vi "Event Log.vi"(8 "Message":string, 9 "Log Event Type":T1, 10 "Event Type":string, 11 "Location":string) -> ()   [LabVIEW 2024, in "Sift TDMS Uploader.lvlib" / "Sift TDMS Uploader.lvclass"]
uses:
  Sift TDMS Uploader.lvclass
  Sift TDMS Uploader.lvclass/Sift TDMS Uploader.ctl
  Log Event Types.ctl
panel:
  in  "error in (no error)":errorcluster
  out "error out":errorcluster
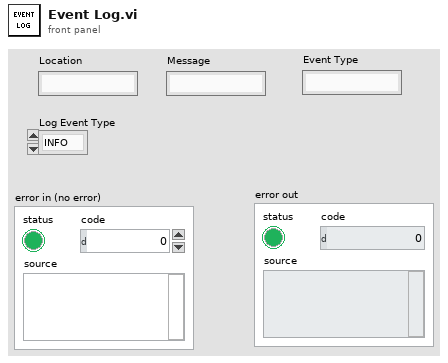
[diagram p1: front panel]
types:
  T1 = typedef "Sift TDMS Uploader.lvlib/Sift TDMS Uploader.lvclass/Log Event Types.ctl" = enum16{"INFO", "WARN", "ERROR"}
  T2 = enum16{"open", "replace", "create", "open or create", "replace or create", "replace or create with confirmation"}
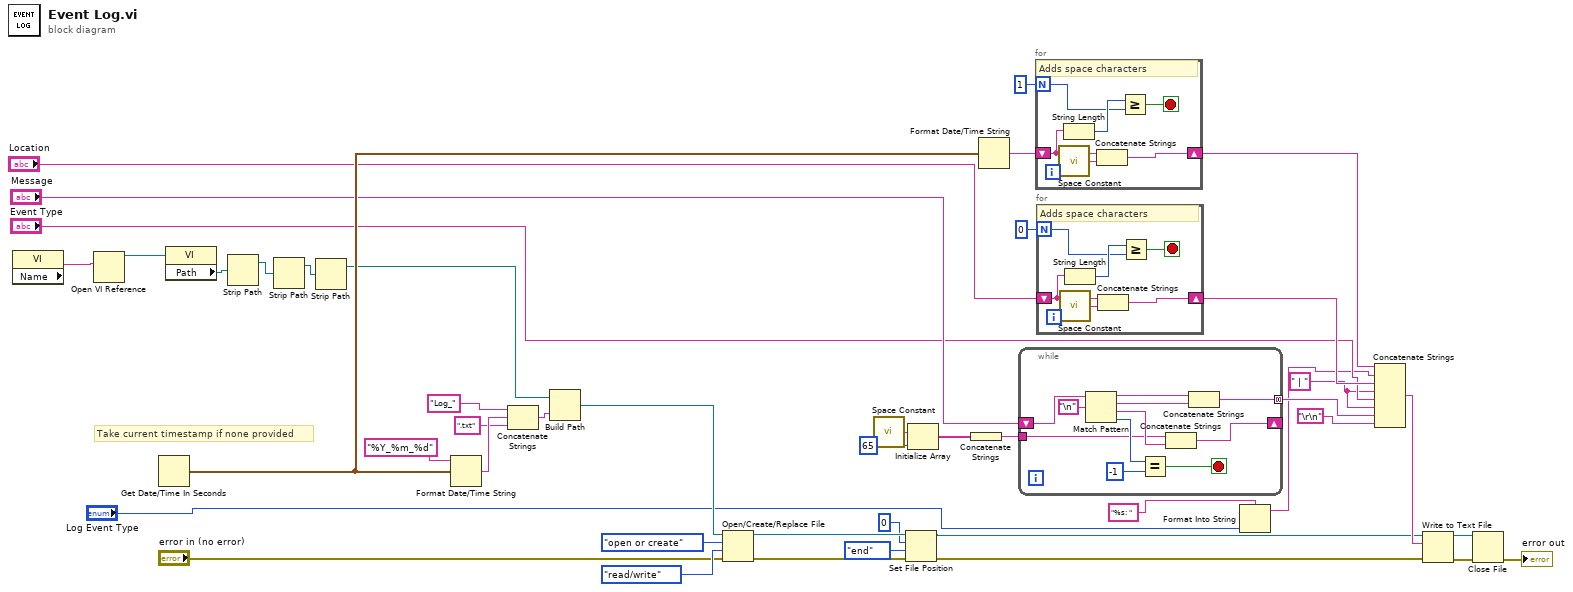
[diagram p0: block diagram]
diagram:
  w7 = " | " ("string")
  # "Take current timestamp if none provided"
  n1 = property class="VI"() -> ("Name"=w13:string)  [unwired: 2 in, 2 out]
  n2 = Open VI Reference(vi path=w13) -> (vi reference=w15:refnum<vi>)  [unwired: 5 in, 1 out]
  n3 = Get Date/Time In Seconds() -> (seconds since 1Jan1904=w17:timestamp)
  n4 = property class="VI"(reference=w15) -> ("Path"=w14:path)  [unwired: 1 in, 2 out]
  n5 = Strip Path(path=w14) -> (stripped path=w6:path)  [unwired: 1 out]
  n6 = Strip Path(path=w6) -> (stripped path=w2:path)  [unwired: 1 out]
  n7 = Strip Path(path=w2) -> (stripped path=w3:path)  [unwired: 1 out]
  n8 = Format Date/Time String(time format string (%c)="%Y_%m_%d", seconds (now)=w17) -> (date/time string=w32:string)  [unwired: 1 in]
  n9 = Concatenate Strings("Log_" ("string"), w32, ".txt" ("string")) -> (w31:string)
  n10 = Build Path(base path=w3, name or relative path=w31) -> (appended path=w18:path)
  n11 = Open/Create/Replace File(file path (use dialog)=w18, error in="error in (no error)", operation (0:open)=T2."open or create", access (0:read/write)=enum16{"read/write", "read-only", "write-only"}."read/write") -> (refnum out=w27:refnum<file>, error out=w28:errorcluster)  [unwired: 2 in, 1 out]
  n12 = call <vilib>:"Space Constant.vi"() -> ("String"=w38:string)
  n13 = Set File Position(offset (in bytes) (0)=i64 0, refnum=w27, from (0:start)=enum16{"start", "end", "current"}."end", error in=w28) -> (refnum out=w19:refnum<file>, error out=w23:errorcluster)
  n14 = Initialize Array(w38, 65 ("dimension size")) -> (w36:string[])
  n15 = Concatenate Strings(w36) -> (w35:string)
  n16 = Format Date/Time String(seconds (now)=w17) -> (date/time string=w41:string)  [unwired: 2 in]
  n17 = while {
    shift-right: [w48] -> _
    shift-left: "Message" -> [w51]
    tunnel: w35 -> [w49]
    tunnel: [w45] -> w9 mode=concatenating
    stop <- w52 stop-if-true
    n18 = Match Pattern(string=w51, regular expression="\n") -> (before substring=w47:string, match substring=w46:string, after substring=w50:string, offset past match=w53:i32)  [unwired: 1 in]
    n19 = Equal?(x=w53, y=-1) -> (x = y?=w52:bool)
    n20 = Concatenate Strings(w49, w50) -> (w48:string)
    n21 = Concatenate Strings(w47, w46) -> (w45:string)
  }
  n22 = for {
    N: 1 -> [w56]
    shift-right: [w58] -> w40
    shift-left: w41 -> [w61]
    stop <- w57 stop-if-true
    # "Adds space characters"
    n23 = call <vilib>:"Space Constant.vi"() -> ("String"=w59:string)
    n24 = String Length(string=w61) -> (length=w60:i32)
    n25 = Concatenate Strings(w61, w59) -> (w58:string)
    n26 = Greater Or Equal?(x=w60, y=w56) -> (x >= y?=w57:bool)
  }
  n27 = for {
    N: 0 -> [w62]
    shift-right: [w64] -> w39
    shift-left: "Location" -> [w67]
    stop <- w63 stop-if-true
    # "Adds space characters"
    n28 = call <vilib>:"Space Constant.vi"() -> ("String"=w65:string)
    n29 = String Length(string=w67) -> (length=w66:i32)
    n30 = Concatenate Strings(w67, w65) -> (w64:string)
    n31 = Greater Or Equal?(x=w66, y=w62) -> (x >= y?=w63:bool)
  }
  n32 = Format Into String(format string="%s: ", "Log Event Type") -> (resulting string=w1:string)  [unwired: 2 in, 1 out]
  n33 = Concatenate Strings(w40, w1, w39, w7, "Event Type", w7, w9, "\r\n") -> (w44:string)
  n34 = Write to Text File(file (use dialog)=w19, text=w44, error in=w23) -> (refnum out=w22:refnum<file>, error out=w21:errorcluster)  [unwired: 1 in, 1 out]
  n35 = Close File(refnum=w22, error in=w21) -> (error out=→"error out":errorcluster)  [unwired: 1 out]
